vi "Get Property Data (Dictionary).vi"(8 "error in":errorcluster, 10 "Property Name":string, 11 "Item Ref in":refnum<data-value>) -> (0 "error out":errorcluster, 3 "Property Value":map{string, string}(c390))   [LabVIEW 2024, in "Config File Parser.lvlib" / "Property.lvclass"]
uses:
  Property.lvclass
  Item/Item.lvclass
  Property Type.ctl
  Property.lvclass/Property.ctl
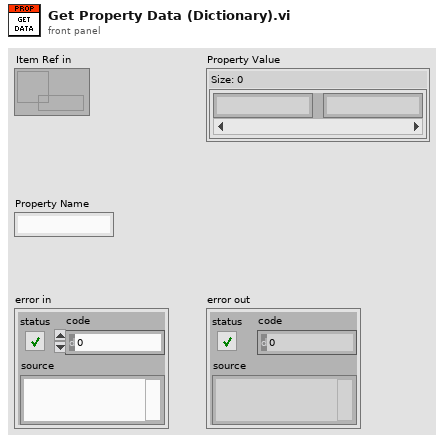
[diagram p1: front panel]
types:
  T1 = typedef "Config File Parser.lvlib/Property.lvclass/Property Type.ctl" = enum16{"Boolean", "Double", "String", "Path", "Dictionary", "DependentFile", "I16", "I32", "I64", "U16", "U32", "U64", "BooleanArray", "DoubleArray", "StringArray", "I16Array", "I32Array", "I64Array", "U16Array", "U32Array", "U64Array", "Variant"}
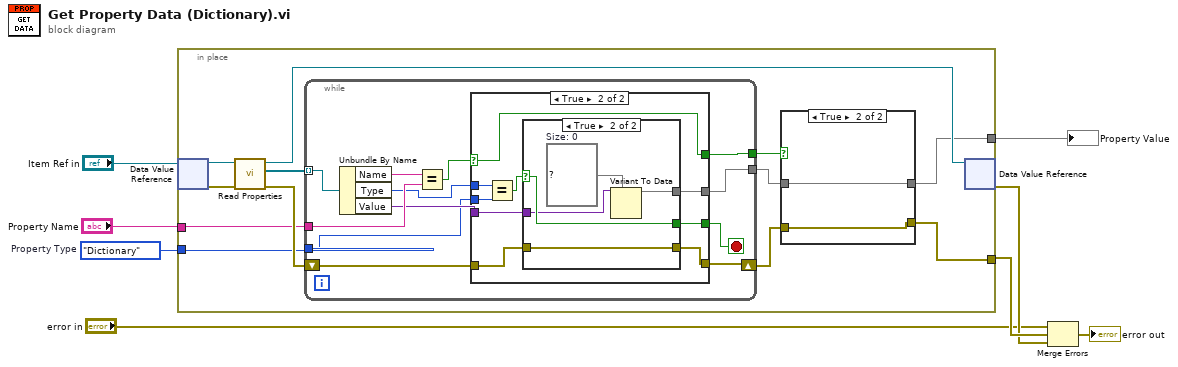
[diagram p0: block diagram]
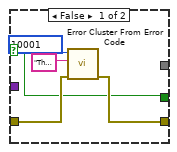
[diagram p3: hidden frame]
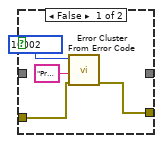
[diagram p4: hidden frame]
diagram:
  w2 = Property_Type."Dictionary"  # Property Type
  n1 = in-place "In Place Element Structure" {
    in-place-border: "Property Name" -> [w15]
    in-place-border: w2 -> [w14]
    in-place-border: [w19] -> w8
    in-place-border: [w10] -> w1
    n2 = in-place-dvr #1("Item Ref in") -> (w16:refnum<class "Item.lvclass">, w20:errorcluster)
    n3 = call-dynamic "Read Properties.vi"("error in (no error)"=w20, "Item in"=w16) -> ("error out"=w18:errorcluster, "Properties"=w9:refnum<class "Property.lvclass">[], "Item out"=w13:refnum<class "Item.lvclass">)  [unwired: 7 in]
    n4 = while {
      tunnel: w15 -> [w28]
      tunnel: w14 -> [w24]
      tunnel: [w25] -> w12
      tunnel: [w23] -> w11
      tunnel: w9 -> [w22] mode=indexing
      shift-right: [w31] -> w17
      shift-left: w18 -> [w32]
      stop <- w21 stop-if-true
      n5 = Unbundle By Name(w22) -> ("Name"=w29:string, "Type"=w26:T1, "Value"=w27:variant)
      n6 = Equal?(x=w29, y=w28) -> (x = y?=w30:bool)
      n7 = case shown="True" w30 {
        selector: w30 -> [w33 w36]
        tunnel: [_ w41] -> w23
        tunnel: w27 -> [_ w40]
        tunnel: w24 -> [_ w38]
        tunnel: w26 -> [_ w39]
        tunnel: [w33 w36] -> w25
        tunnel: [w33 w35] -> w21
        tunnel: w32 -> [w34 w43]
        tunnel: [w34 w42] -> w31
        frame False {
        }
        frame True {
          n8 = Equal?(x=w39, y=w38) -> (x = y?=w37:bool)
          n9 = case shown="True" w37 {
            selector: w37 -> [w44 w51]
            tunnel: [_ w52] -> w41
            tunnel: w40 -> [_ w50]
            tunnel: [w44 w51] -> w35
            tunnel: w43 -> [w48 w53]
            tunnel: [w47 w53] -> w42
            frame False {
              n10 = call <vilib>:"Error Cluster From Error Code.vi"("error in (no error)"=w48, "error message (\"\")"="The selected type is incompatible with the chosen property", "error code (0)"=10001) -> ("error out"=w47:errorcluster)  [unwired: 6 in]
            }
            frame True {
              w49 = map{string, string} {}  # Size: 0
              n11 = Variant To Data(type=w49, Variant=w50) -> (data=w52:map{string, string})  [unwired: 1 in, 1 out]
            }
          }
        }
      }
    }
    n12 = case shown="True" w12 {
      tunnel: w11 -> [_ w58]
      tunnel: [_ w58] -> w10
      tunnel: [w57 w59] -> w19
      tunnel: w17 -> [w56 w59]
      frame False {
        n13 = call <vilib>:"Error Cluster From Error Code.vi"("error in (no error)"=w56, "error message (\"\")"="Property does not exist", "error code (0)"=10002) -> ("error out"=w57:errorcluster)  [unwired: 6 in]
      }
      frame True {
      }
    }
    n14 = in-place-dvr #1(w13) -> (w7:errorcluster)  [unwired: 1 out]
  }
  "Property Value" <- w1
  n15 = Merge Errors("error in", w8, w7) -> (→"error out":errorcluster)
